vi "DataToRead.vi"(8 "error in (no error)":errorcluster, 11 "BaseReader in":refnum<class "BaseReader.lvclass">) -> (0 "error out":errorcluster, 2 "Data available?":bool, 3 "BaseReader out":refnum<class "BaseReader.lvclass">)   [LabVIEW 2025, in "BaseReader.lvclass"]
doc: "Returns TRUE if there is any data to read from the remote host"
uses:
  BaseReader.lvclass
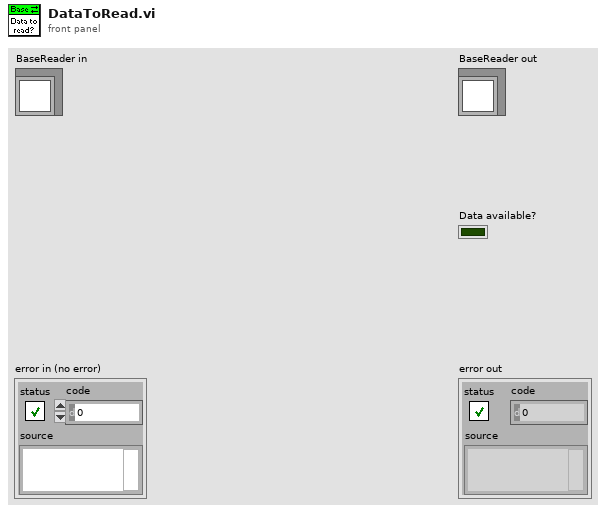
[diagram p1: front panel]
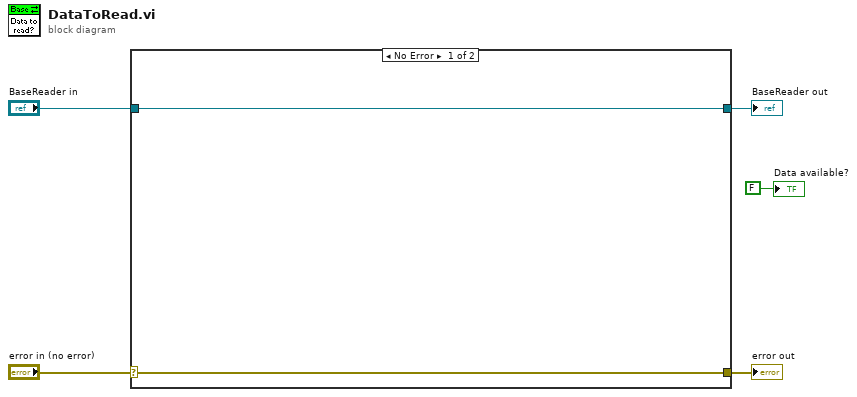
[diagram p0: block diagram]
diagram:
  n1 = case shown="No Error" "error in (no error)" {
    selector: "error in (no error)" -> [w6 w9]
    tunnel: [w6 w9] -> w4
    tunnel: [w7 w8] -> w2
    tunnel: "BaseReader in" -> [w7 w8]
    frame No Error {
    }
    frame Error {
    }
  }
  "error out" <- w4
  "BaseReader out" <- w2
  "Data available?" <- FALSE
